vi "Write Time Stamp.vi"(7 "field name":string="timeStamp", 8 "error in":errorcluster, 9 "user tag in":i32, 10 "timestamp in":timestamp, 11 "PV Data in":refnum<class "PV Data.lvclass">) -> (0 "error out":errorcluster, 1 "user tag out":i32, 2 "timestamp out":timestamp, 3 "PV Data out":refnum<class "PV Data.lvclass">)   [LabVIEW 2020, in "PV Access.lvlib" / "PV Data.lvlib" / "PV Data.lvclass"]
uses:
  PV Data.lvclass
  PV Access.lvlib
  PV Data.lvlib
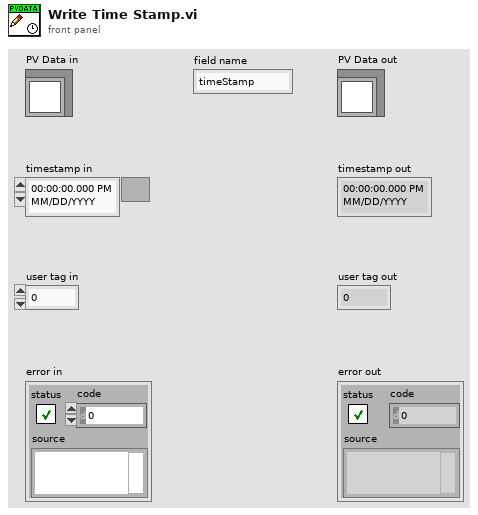
[diagram p1: front panel]
types:
  T1 = typedef "PV Access.lvlib/PV Data.lvlib/EPICS Time Stamp.ctl" = cluster{"secondsPastEpoch":i64, "nanoseconds":i32, "userTag":i32}
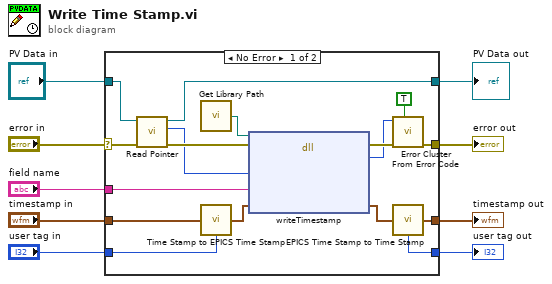
[diagram p0: block diagram]
diagram:
  n1 = case shown="No Error" "error in" {
    selector: "error in" -> [w21 w30]
    tunnel: [w22 w30] -> w9
    tunnel: "PV Data in" -> [w19 w29]
    tunnel: [w17 w29] -> w6
    tunnel: "field name" -> [w16 _]
    tunnel: "timestamp in" -> [w15 w28]
    tunnel: "user tag in" -> [w14 w27]
    tunnel: [w11 w28] -> w2
    tunnel: [w10 w27] -> w1
    frame No Error {
      n2 = call-dynamic "Read Pointer.vi"("error in (no error)"=w21, "Pointer Base in"=w19) -> ("error out"=w20:errorcluster, "Pointer"=w18:i64, "Pointer Base out"=w17:refnum<class "PV Data.lvclass">)  [unwired: 7 in]
      n3 = call "Get Library Path.vi"() -> ("Path"=w26:path)  [unwired: 1 in]
      n4 = call "Time Stamp to EPICS Time Stamp.vi"("time stamp"=w15, "user tag"=w14) -> ("EPICS time stamp"=w13:T1)
      n5 = dll-call lib="?" fn="writeTimestamp"(path in=w26, error in=w20, "value"=w18, "field_name"=w16, "timestamp"=w13) -> (error out=w24:errorcluster, "err_code"=w23:i32, "timestamp"=w12:T1)  [unwired: 3 in, 1 out]
      n6 = call <vilib>:"Error Cluster From Error Code.vi"("show call chain? (False)"=TRUE, "error in (no error)"=w24, "error code (0)"=w23) -> ("error out"=w22:errorcluster)  [unwired: 6 in]
      n7 = call "EPICS Time Stamp to Time Stamp.vi"("EPICS time stamp"=w12) -> ("user tag"=w10:i32, "time stamp"=w11:timestamp)
    }
    frame Error {
    }
  }
  "error out" <- w9
  "PV Data out" <- w6
  "timestamp out" <- w2
  "user tag out" <- w1
